vi "close connection.vi"(8 "error in (no error)":errorcluster, 11 "Class 4 in":refnum<class "Class 4.lvclass">) -> (0 "error out":errorcluster, 3 "Class 4 out":refnum<class "Class 4.lvclass">)   [LabVIEW 2013, in "Class 4.lvclass"]
doc: "Visa-Verbindung mit dem Gerät schliessen."
uses:
  Class 4.lvclass
  DeviceInterface/DeviceInterface.lvclass
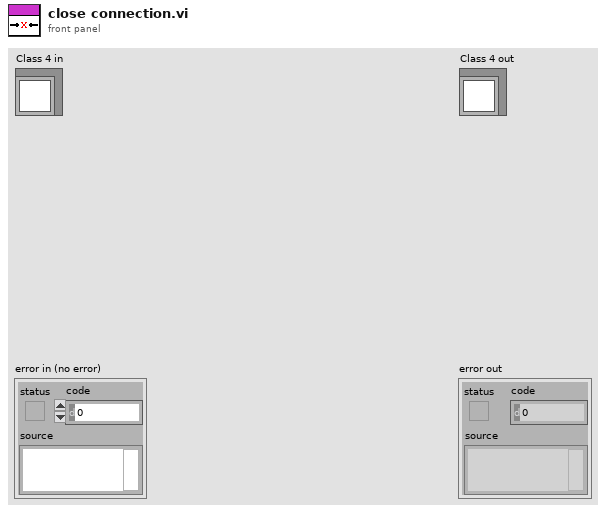
[diagram p1: front panel]
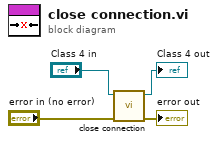
[diagram p0: block diagram]
diagram:
  n1 = call-parent "close connection.vi"("error in (no error)"="error in (no error)", "DeviceInterface in"="Class 4 in") -> ("error out"=→"error out":errorcluster, "DeviceInterface out"=→"Class 4 out":refnum<class "Class 4.lvclass">)  [unwired: 8 in]
